vi "Serial Read.vi"(8 "error in (no error)":errorcluster, 9 "timeout (ms)":i32, 10 "bytes to read":i32, 11 "VISA resource":refnum<visa-resource-name>) -> (0 "error out":errorcluster, 1 "timed out?":bool, 3 "data":u8[](array[numeric]))   [LabVIEW 2015, in "SubVIs.lvlib" / "Serial Shared Components.lvlib"]
doc: "Performs a read on the serial port."
uses:
  <vilib>/Modbus/subvis/Protocol/Serial/Serial Shared Components/Serial Shared Components.lvlib
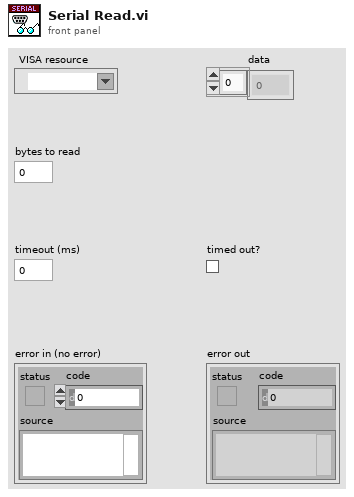
[diagram p1: front panel]
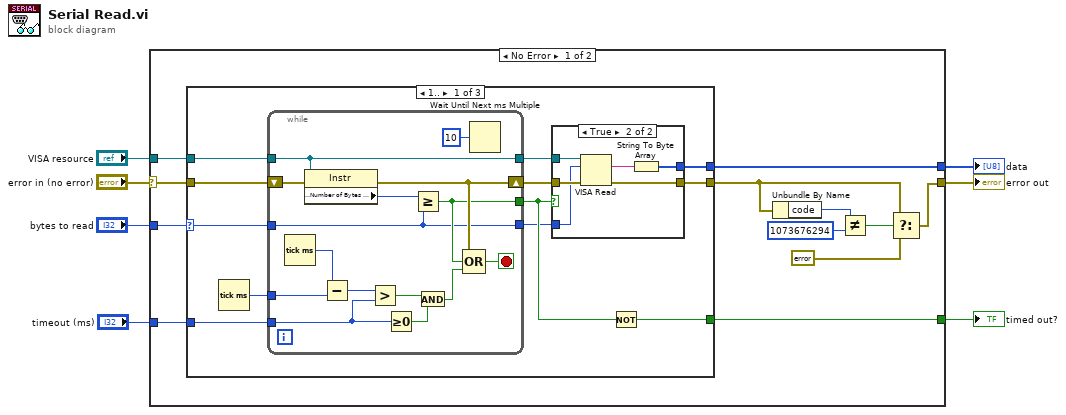
[diagram p0: block diagram]
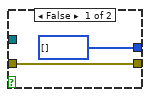
[diagram p2: hidden frame]
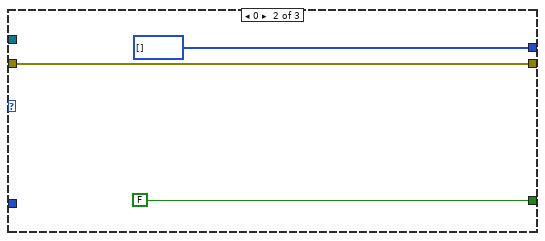
[diagram p3: hidden frame]
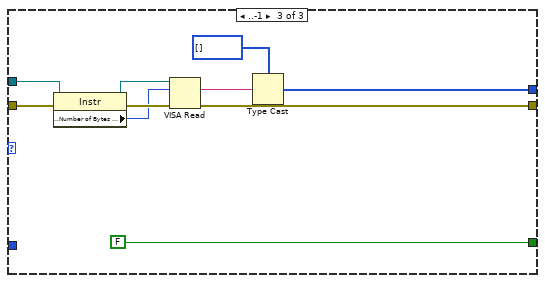
[diagram p4: hidden frame]
diagram:
  n1 = case shown="No Error" "error in (no error)" {
    selector: "error in (no error)" -> [w8 w68]
    tunnel: "bytes to read" -> [w19 _]
    tunnel: "timeout (ms)" -> [w18 _]
    tunnel: "VISA resource" -> [w17 _]
    tunnel: [w16 _] -> w4
    tunnel: [w15 _] -> w3
    tunnel: [w9 w68] -> w2
    frame No Error {
      n2 = case shown="1.." w19 {
        selector: w19 -> [w26 _ _]
        tunnel: w18 -> [w24 _ _]
        tunnel: w8 -> [w30 w57 w67]
        tunnel: w17 -> [w25 _ w66]
        tunnel: [w28 w57 w62] -> w11
        tunnel: [w27 u8[] [] ("data") w60] -> w16
        tunnel: [w22 FALSE FALSE] -> w15
        frame 1.. {
          n3 = Tick Count (ms)() -> (millisecond timer value=w31:u32)
          n4 = while {
            tunnel: w31 -> [w48]
            shift-right: [w52] -> w29
            shift-left: w30 -> [w54]
            tunnel: w26 -> [w41]
            tunnel: w25 -> [w42]
            tunnel: [w51] -> w23
            tunnel: w24 -> [w44]
            tunnel: [w42] -> w21
            tunnel: [w41] -> w20
            stop <- w50 stop-if-true
            n5 = Tick Count (ms)() -> (millisecond timer value=w49:u32)
            n6 = property class="Instr"(reference=w42, error in=w54) -> (error out=w52:errorcluster, "Serial Settings:Number of Bytes at Serial Port"=w53:u32)  [unwired: 1 out]
            n7 = Subtract(x=w49, y=w48) -> (x-y=w46:u32)
            n8 = Greater?(x=w46, y=w44) -> (0:w45:bool)
            n9 = Greater Or Equal To 0?(x=w44) -> (x >= 0?=w43:bool)
            n10 = Greater Or Equal?(x=w53, y=w41) -> (x >= y?=w51:bool)
            n11 = And(x=w45, y=w43) -> (x .and. y?=w47:bool)
            n12 = Compound Arithmetic op=OR(w52, w51, w47) -> (w50:bool)
            n13 = Wait Until Next ms Multiple(millisecond multiple=u32 10) -> ()  [unwired: 1 out]
          }
          n14 = case shown="True" w23 {
            tunnel: w29 -> [w32 w39]
            tunnel: [w32 w38] -> w28
            tunnel: [u8[] [] ("data") w37] -> w27
            tunnel: w21 -> [_ w35]
            tunnel: w20 -> [_ w34]
            frame False {
            }
            frame True {
              n15 = VISA Read(VISA resource name=w35, byte count=w34, error in (no error)=w39) -> (read buffer=w36:string, error out=w38:errorcluster)  [unwired: 2 out]
              n16 = String To Byte Array(string=w36) -> (unsigned byte array=w37:u8[])
            }
          }
          n17 = Not(x=w23) -> (.not. x?=w22:bool)
        }
        frame 0 {
        }
        frame ..-1 {
          n18 = property class="Instr"(reference=w66, error in=w67) -> (reference out=w64:refnum<visa-resource-name>, error out=w65:errorcluster, "Serial Settings:Number of Bytes at Serial Port"=w63:u32)
          n19 = VISA Read(VISA resource name=w64, byte count=w63, error in (no error)=w65) -> (read buffer=w59:string, error out=w62:errorcluster)  [unwired: 2 out]
          n20 = Type Cast(type=u8[] [] ("data"), x=w59) -> (*(type *) &x=w60:u8[])
        }
      }
      n21 = Unbundle By Name(w11) -> ("code"=w14:i32)
      n22 = Not Equal?(x=w14, y=1073676294) -> (x != y?=w12:bool)
      n23 = Select(t=w11, s=w12, f=errorcluster {"status"=FALSE, "code"=0, "source"=""}) -> (s? t:f=w9:errorcluster)
    }
    frame Error {
    }
  }
  "error out" <- w2
  "data" <- w4
  "timed out?" <- w3
